vi "140文件解析测试.vi"() -> ()   [LabVIEW 2018]
panel:
  out "错误输出":errorcluster
  out "140二维码":string
  out "压机旋铆位移压力图_1":cluster{dbl[], dbl[]}(graph)
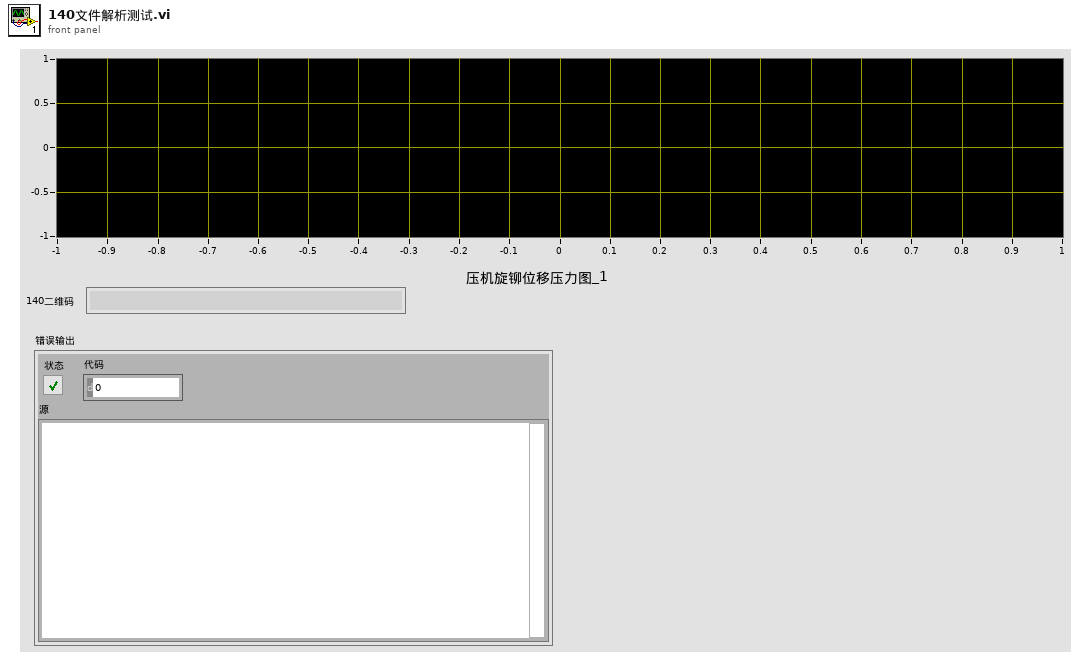
[diagram p1: front panel]
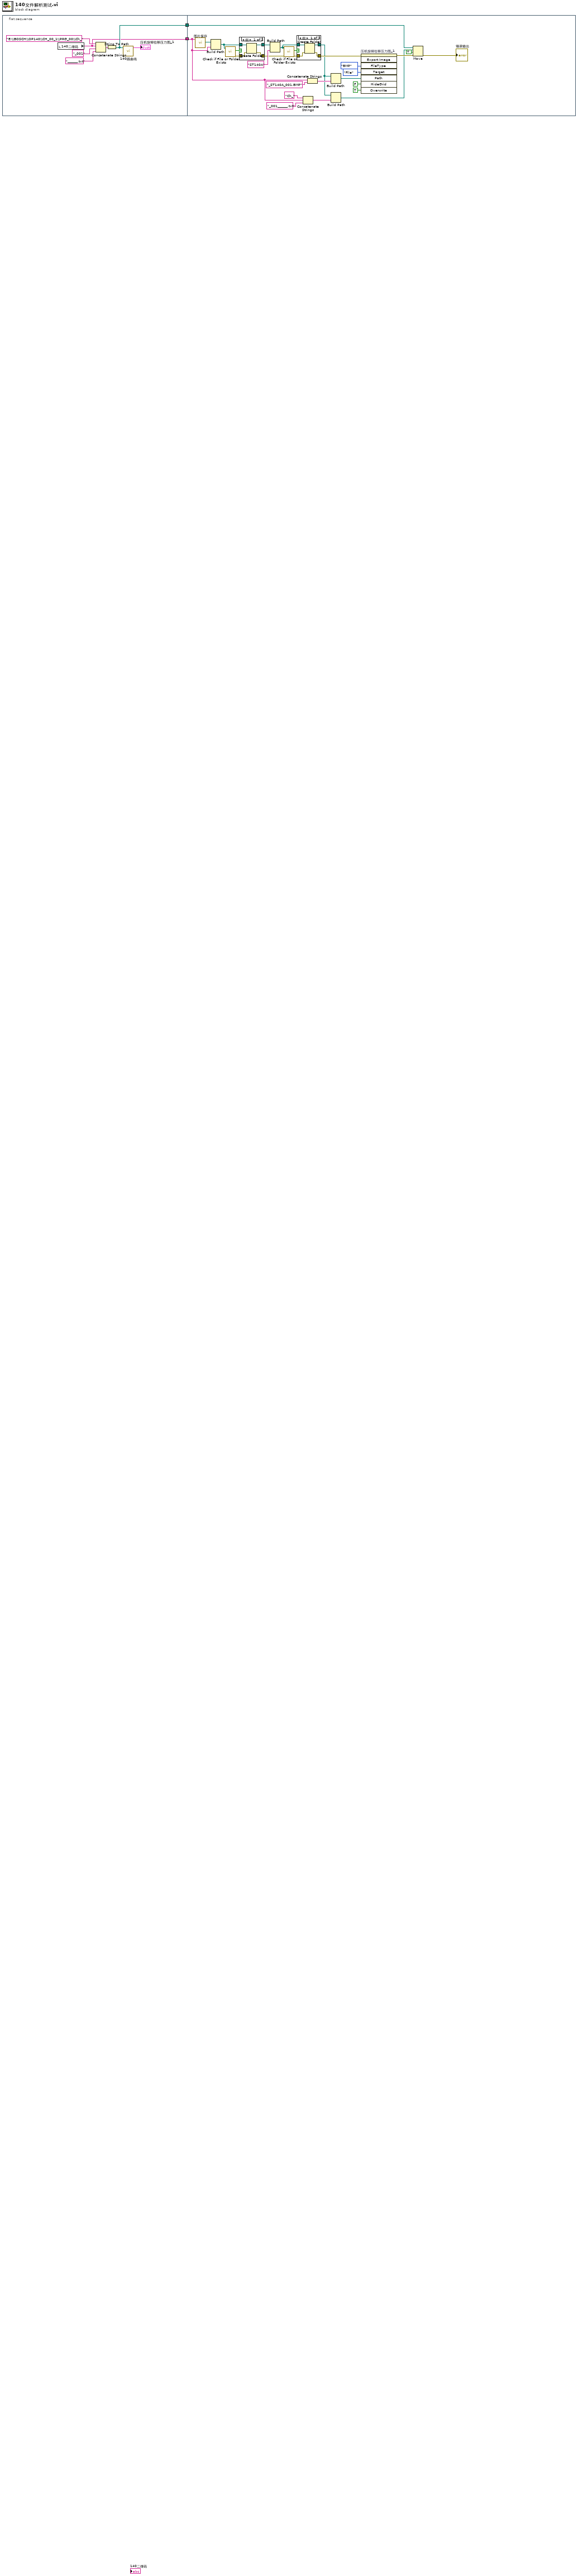
[diagram p0: block diagram]
diagram:
  n1 = flat-sequence {
    tunnel: [w3] -> w2
    tunnel: [w4] -> w1
    tunnel: w2 -> [w15]
    tunnel: w1 -> [w18]
    frame #0 {
      n2 = local read "140二维码"() -> (w3:string)
      n3 = Concatenate Strings("E:\\BOSCH\\OP140\\CH_00_1\\PRG_00\\Ch_", w3, "_001", "______.txt" ("字符串")) -> (w7:string)
      n4 = String To Path(string=w7) -> (path=w4:path)
      n5 = call "140画曲线.vi"("文件（使用对话框）"=w4) -> ("压机旋铆位移压力图"=→"压机旋铆位移压力图_1":cluster{dbl[], dbl[]})  [unwired: 10 in]
    }
    frame #1 {
      n6 = call "图片保存.vi"("一维码"=w15) -> ("dup path"=w37:path)  [unwired: 9 in, 1 out]
      n7 = Build Path(base path=w37, name or relative path=w15) -> (appended path=w36:path)
      n8 = call <vilib>:"Check if File or Folder Exists.vi"("path"=w36) -> ("error out"=w34:errorcluster, "file or folder exists?"=w35:bool)  [unwired: 8 in, 1 out]
      n9 = case shown="假" w35 {
        tunnel: w36 -> [w47 w49]
        tunnel: [w46 w49] -> w30
        tunnel: w34 -> [w45 w48]
        tunnel: [w44 w48] -> w28
        frame False {
          n10 = Create Folder(path (use dialog)=w47, error in=w45) -> (created path=w46:path, error out=w44:errorcluster)  [unwired: 1 in, 1 out]
        }
        frame True {
        }
      }
      n11 = Build Path(base path=w30, name or relative path="ST140A" ("名称或相对路径")) -> (appended path=w31:path)
      n12 = call <vilib>:"Check if File or Folder Exists.vi"("error in (no error)"=w28, "path"=w31) -> ("error out"=w32:errorcluster, "file or folder exists?"=w33:bool)  [unwired: 7 in, 1 out]
      n13 = case shown="假" w33 {
        tunnel: w31 -> [w41 w43]
        tunnel: [w40 w43] -> w17
        tunnel: w32 -> [w39 w42]
        tunnel: [w38 w42] -> w27
        frame False {
          n14 = Create Folder(path (use dialog)=w41, error in=w39) -> (created path=w40:path, error out=w38:errorcluster)  [unwired: 1 in, 1 out]
        }
        frame True {
        }
      }
      n15 = Concatenate Strings("Ch_" ("字符串"), w15, "_001______.txt" ("字符串")) -> (w13:string)
      n16 = Concatenate Strings(w15, "_ST140A_001.BMP" ("字符串")) -> (w21:string)
      n17 = Build Path(base path=w17, name or relative path=w21) -> (appended path=w20:path)
      n18 = Build Path(base path=w17, name or relative path=w13) -> (appended path=w12:path)
      n19 = invoke on="压机旋铆位移压力图_1" class="XYGraph (严格)" method="Export Image"(error in=w27, "FileType"=enum32{"BMP", "EPS", "EMF", "PICT"}."BMP" ("文件类型"), "Target"=enum32{"File", "Clipboard"}."File" ("目标"), "Path"=w20, "HideGrid"=FALSE ("隐藏网格"), "Overwrite"=TRUE ("始终覆盖")) -> (error out=w19:errorcluster)  [unwired: 2 in, 7 out]
      n20 = Move(source path=w18, error in=w19, 9:TRUE ("覆盖(F)"), 10:w12) -> (error out=→"错误输出":errorcluster)  [unwired: 1 in, 2 out]
    }
  }
